vi "Horizontal Concat Image Data (ARGB).vi"(1 "B":u8[][](array[numeric]), 2 "A":u8[][](array[numeric])) -> (0 "A Horizontal Concatinated with B":u8[][](array[numeric]))   [LabVIEW 2020, in "image.lvlib"]
doc: "Horizontally Concatinate Image Data Arrays."
uses:
  image.lvlib
  626c57e5-3d65-474e-90f8-581bf1c8691a.vi
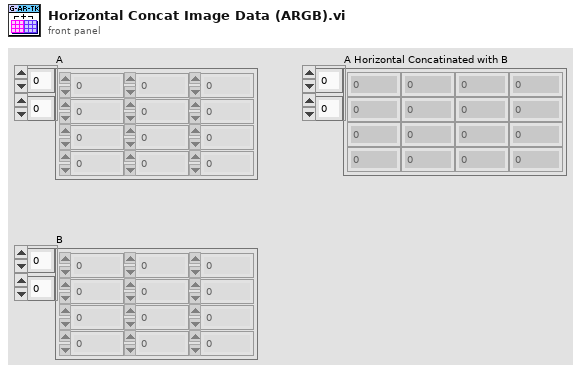
[diagram p1: front panel]
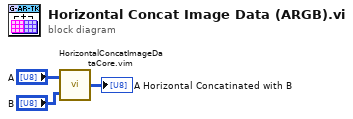
[diagram p0: block diagram]
diagram:
  n1 = call "HorizontalConcatImageDataCore.vim"("B"="B", "A"="A") -> ("A Horizontal Concatinated with B"=→"A Horizontal Concatinated with B":u8[][])
